vi "DSF.Shared.Configuration.Framework.Validate.vi"(8 "error in (no error)":errorcluster, 11 "Framework Configuration in":refnum<class "DSF.Shared.Configuration.Framework.lvclass">) -> (0 "error out":errorcluster, 3 "Framework Configuration out":refnum<class "DSF.Shared.Configuration.Framework.lvclass">)   [LabVIEW 2016, in "DSF.Shared.lvlib" / "DSF.Shared.Configuration.Framework.lvclass"]
uses:
  DSF.Shared.Configuration.Framework.lvclass
  DSF.Shared.Configuration.Framework.lvclass/DSF.Shared.Configuration.Framework.ctl
  Plugin/DSF.Shared.Configuration.Plugin.lvclass
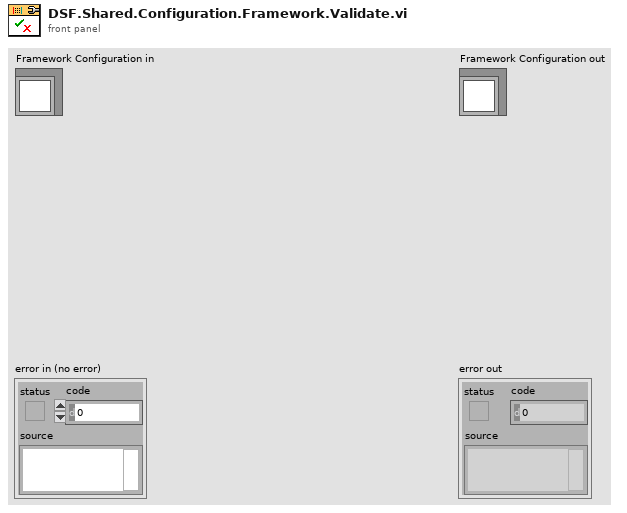
[diagram p1: front panel]
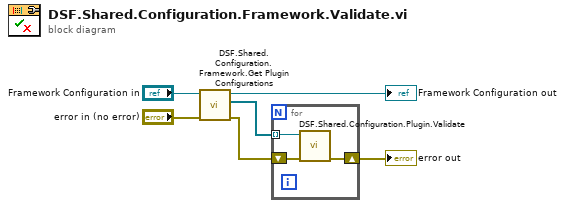
[diagram p0: block diagram]
diagram:
  n1 = call "DSF.Shared.Configuration.Framework.Get Plugin Configurations.vi"("error in (no error)"="error in (no error)", "Framework Configuration in"="Framework Configuration in") -> ("error out"=w3:errorcluster, "Plugin Configurations"=w4:refnum<class "DSF.Shared.Configuration.Plugin.lvclass">[], "Framework Configuration out"=→"Framework Configuration out":refnum<class "DSF.Shared.Configuration.Framework.lvclass">)  [unwired: 7 in]
  n2 = for {
    tunnel: w4 -> [w9] mode=indexing
    shift-right: [w7] -> w1
    shift-left: w3 -> [w8]
    n3 = call "DSF.Shared.Configuration.Plugin.Validate.vi"("error in (no error)"=w8, "Plugin Configuration in"=w9) -> ("error out"=w7:errorcluster)  [unwired: 8 in, 1 out]
  }
  "error out" <- w1
